vi "SpawnFood.vi"(9 "X Position":i32, 10 "Y Position":i32, 11 "Level input":u32[][](array[colorbox])) -> (3 "Level output":u32[][](array[colorbox]))   [LabVIEW 2021]
uses:
  GlobalVariables/Board_Colors.vi
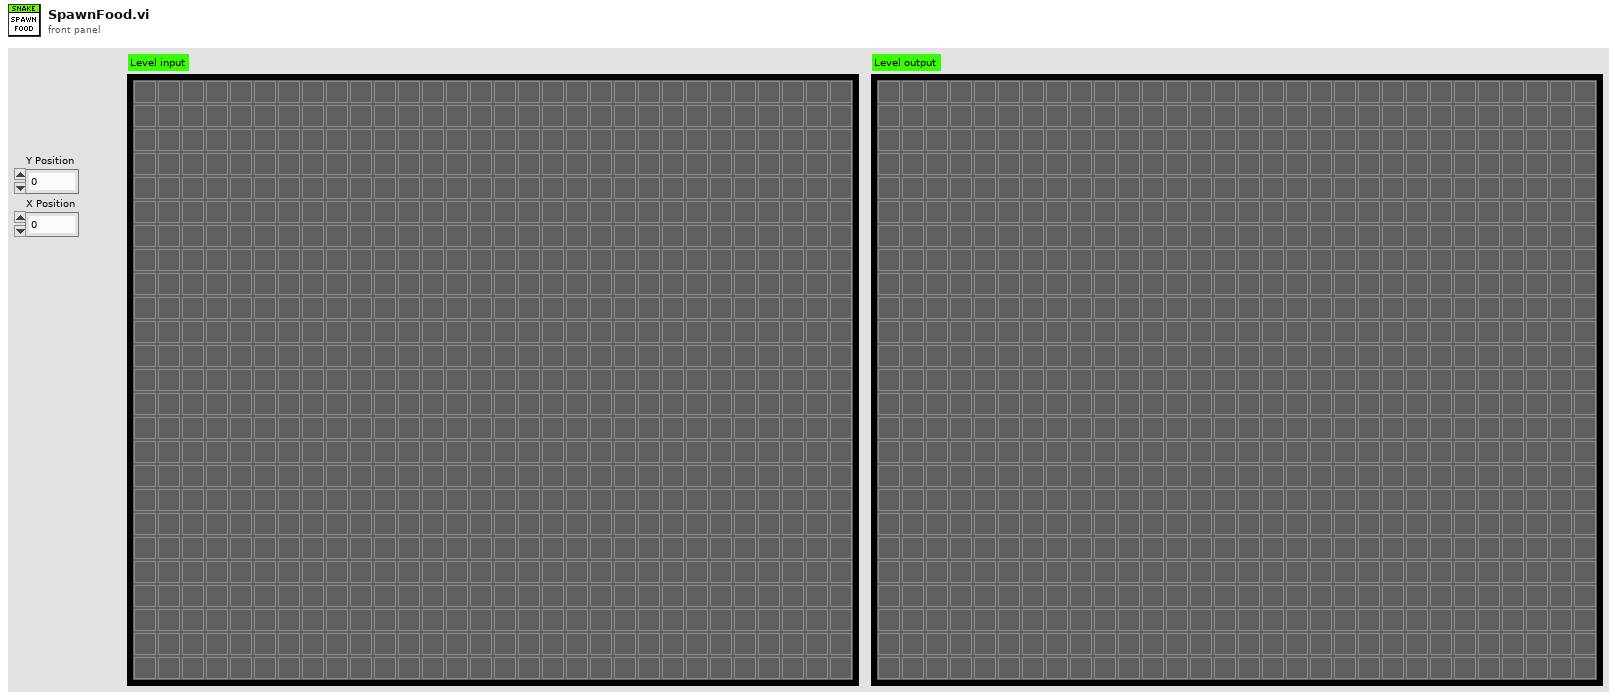
[diagram p1: front panel]
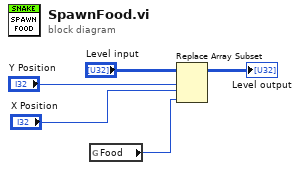
[diagram p0: block diagram]
diagram:
  n1 = global read "Board_Colors.vi" "Food"() -> (w1:u32)
  n2 = Replace Array Subset(array="Level input", new element=w1, index (row)="Y Position", index (col)="X Position") -> (→"Level output":u32[][])
